vi "sun_bresenham.vi"(10 "stop":cluster{"x2":dbl, "y2":dbl}, 11 "start":cluster{"x1":dbl, "y1":dbl}) -> ()   [LabVIEW 2019]
panel:
  out "dy":dbl
  out "dx":dbl
  out "error":i32
  out "swapped":bool
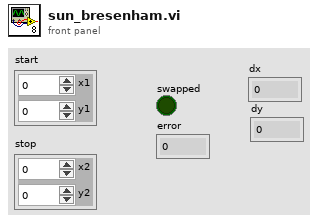
[diagram p1: front panel]
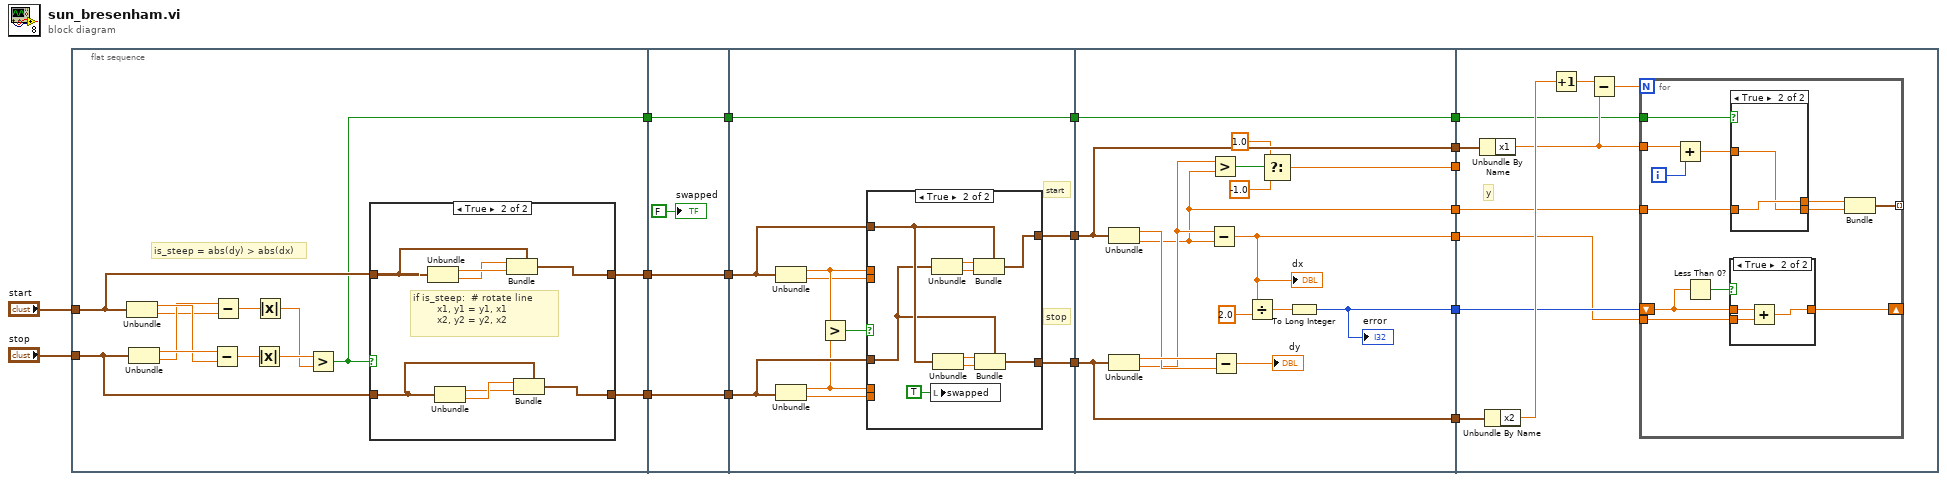
[diagram p0: block diagram]
diagram:
  n1 = flat-sequence {
    tunnel: "start" -> [w23]
    tunnel: "stop" -> [w22]
    tunnel: [w21] -> w16
    tunnel: [w20] -> w14
    tunnel: [w19] -> w6
    tunnel: w16 -> [w45]
    tunnel: [w45] -> w15
    tunnel: w14 -> [w44]
    tunnel: [w44] -> w13
    tunnel: w6 -> [w42]
    tunnel: [w42] -> w3
    tunnel: w15 -> [w54]
    tunnel: w13 -> [w53]
    tunnel: [w48] -> w12
    tunnel: [w47] -> w11
    tunnel: [w46] -> w4
    tunnel: w3 -> [w46]
    tunnel: w12 -> [w82]
    tunnel: w11 -> [w81]
    tunnel: [w82] -> w10
    tunnel: [w81] -> w9
    tunnel: [w71] -> w8
    tunnel: [w70] -> w7
    tunnel: [w69] -> w5
    tunnel: w4 -> [w69]
    tunnel: [w68] -> w2
    tunnel: [w67] -> w1
    tunnel: w10 -> [w92]
    tunnel: w9 -> [w91]
    tunnel: w8 -> [_]
    tunnel: w7 -> [w85]
    tunnel: w5 -> [w86]
    tunnel: w2 -> [w84]
    tunnel: w1 -> [w83]
    frame #0 {
      # "is_steep = abs(dy) > abs(dx)"
      n2 = Unbundle(w23) -> ("x1"=w30:dbl, "y1"=w28:dbl)
      n3 = Unbundle(w22) -> ("x2"=w31:dbl, "y2"=w29:dbl)
      n4 = Subtract(x=w31, y=w30) -> (x-y=w26:dbl)
      n5 = Subtract(x=w29, y=w28) -> (x-y=w27:dbl)
      n6 = Absolute Value(x=w26) -> (abs(x)=w25:dbl)
      n7 = Absolute Value(x=w27) -> (abs(x)=w24:dbl)
      n8 = Greater?(x=w25, y=w24) -> (0:w19:bool)
      n9 = case shown="True" w19 {
        tunnel: w23 -> [w33 w35]
        tunnel: w22 -> [w32 w34]
        tunnel: [w32 w37] -> w20
        tunnel: [w33 w36] -> w21
        frame False {
        }
        frame True {
          # "if is_steep:  # rotate line\n        x1, y1 = y1, x1\n        x2, y2 = y2, x2"
          n10 = Unbundle(w35) -> ("x1"=w41:dbl, "y1"=w40:dbl)
          n11 = Unbundle(w34) -> ("x2"=w38:dbl, "y2"=w39:dbl)
          n12 = Bundle(cluster=w35, "x1"=w40, "y1"=w41) -> (w36:cluster{"x1":dbl, "y1":dbl})
          n13 = Bundle(cluster=w34, "x2"=w39, "y2"=w38) -> (w37:cluster{"x2":dbl, "y2":dbl})
        }
      }
    }
    frame #1 {
      "swapped" <- FALSE
    }
    frame #2 {
      # "stop"
      # "start"
      n14 = Unbundle(w54) -> ("x1"=w52:dbl, "y1"=w50:dbl)
      n15 = Unbundle(w53) -> ("x2"=w51:dbl, "y2"=w49:dbl)
      n16 = Greater?(x=w52, y=w51) -> (0:w55:bool)
      n17 = case shown="True" w55 {
        tunnel: w54 -> [w57 w59]
        tunnel: w53 -> [w56 w58]
        tunnel: w52 -> [_ _]
        tunnel: w51 -> [_ _]
        tunnel: w50 -> [_ _]
        tunnel: w49 -> [_ _]
        tunnel: [w56 w60] -> w47
        tunnel: [w57 w63] -> w48
        frame False {
        }
        frame True {
          n18 = local write "swapped"(TRUE ("swapped")) -> ()
          n19 = Unbundle(w58) -> ("x2"=w65:dbl, "y2"=w64:dbl)
          n20 = Unbundle(w59) -> ("x1"=w61:dbl, "y1"=w62:dbl)
          n21 = Bundle(cluster=w59, "x1"=w65, "y1"=w64) -> (w63:cluster{"x1":dbl, "y1":dbl})
          n22 = Bundle(cluster=w58, "x2"=w61, "y2"=w62) -> (w60:cluster{"x2":dbl, "y2":dbl})
        }
      }
    }
    frame #3 {
      n23 = Unbundle(w82) -> ("x1"=w79:dbl, "y1"=w70:dbl)
      n24 = Unbundle(w81) -> ("x2"=w80:dbl, "y2"=w75:dbl)
      n25 = Subtract(x=w75, y=w70) -> (x-y=w67:dbl)
      "dx" <- w67
      n26 = Greater?(x=w75, y=w70) -> (0:w74:bool)
      n27 = Subtract(x=w80, y=w79) -> (x-y=→"dy":dbl)
      n28 = Divide(x=w67, y=2.0) -> (x/y=w77:dbl)
      n29 = Select(t=1.0, s=w74, f=-1.0) -> (s? t:f=w71:dbl)
      n30 = To Long Integer(number=w77) -> (32bit integer=w68:i32)
      "error" <- w68
    }
    frame #4 {
      # "y"
      n31 = Unbundle By Name(w92) -> ("x1"=w87:dbl)
      n32 = Unbundle By Name(w91) -> ("x2"=w90:dbl)
      n33 = Increment(x=w90) -> (x+1=w89:dbl)
      n34 = Subtract(x=w89, y=w87) -> (x-y=w88:dbl)
      n35 = for {
        N: w88 -> [_]
        tunnel: w87 -> [w103]
        tunnel: w86 -> [w100]
        tunnel: w85 -> [w102]
        tunnel: [w97] -> _ mode=indexing
        shift-right: [w95] -> _
        shift-left: w84 -> [w93]
        tunnel: w83 -> [w96]
        i -> [w104]
        n36 = Add(x=w103, y=w104) -> (x+y=w101:dbl)
        n37 = Less Than 0?(x=w93) -> (x < 0?=w94:bool)
        n38 = case shown="True" w94 {
          tunnel: w93 -> [w105 w108]
          tunnel: w96 -> [_ w107]
          tunnel: [w105 w106] -> w95
          frame False {
          }
          frame True {
            n39 = Add(x=w108, y=w107) -> (x+y=w106:dbl)
          }
        }
        n40 = case shown="True" w100 {
          tunnel: w102 -> [w109 w112]
          tunnel: w101 -> [w110 w111]
          tunnel: [w110 w112] -> w99
          tunnel: [w109 w111] -> w98
          frame False {
          }
          frame True {
          }
        }
        n41 = Bundle("y1"=w99, "y1"=w98) -> (w97:cluster{"y1":dbl, "y1":dbl})  [unwired: 1 in]
      }
    }
  }
